vi "exercice5.vi"() -> ()   [LabVIEW 2020]
uses:
  <vilib>/express/express analysis/Spectral/Block/exnSpectralBlock spectral measurements RMS poly.vi
  <vilib>/express/express analysis/Spectral/Block/exnSpectralBlock spectral measurements RMS WFM.vi
  <vilib>/express/express analysis/Spectral/XNode/ExpressSpectralMeasurementsBlockNode.xnode
  <vilib>/measure/NI_MABase.lvlib
panel:
  out "dsa 1st rectangular":cluster{"f0":dbl, "df":dbl, "magnitude":dbl[]}(graph)
  out "dsa 1st hunning":cluster{"f0":dbl, "df":dbl, "magnitude":dbl[]}(graph)
  out "time domain 1st":waveform(dbl)(graph)
  out "k2":dbl
  out "k1":dbl
  out "tw":dbl
  out "freauency resolution":dbl
  in  "N":dbl
  in  "fs":dbl
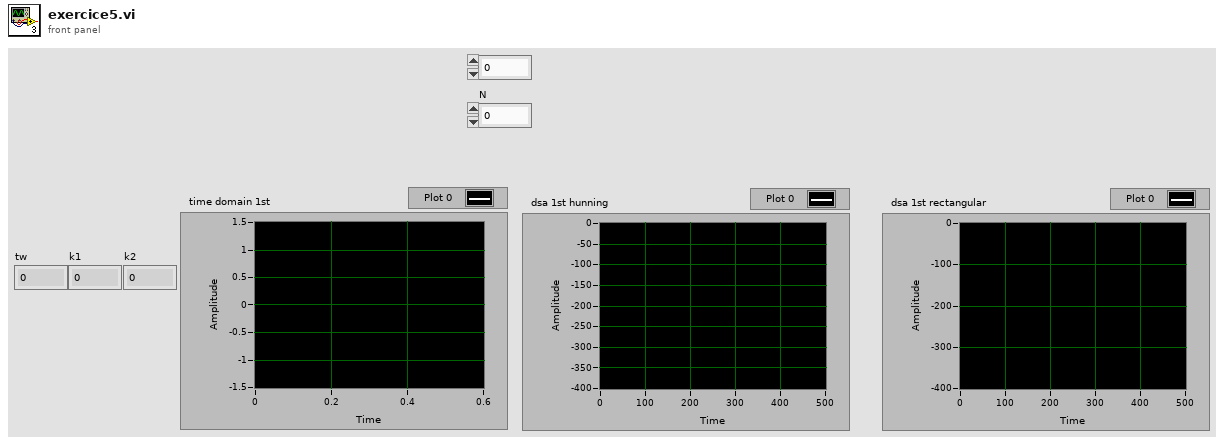
[diagram p1: front panel]
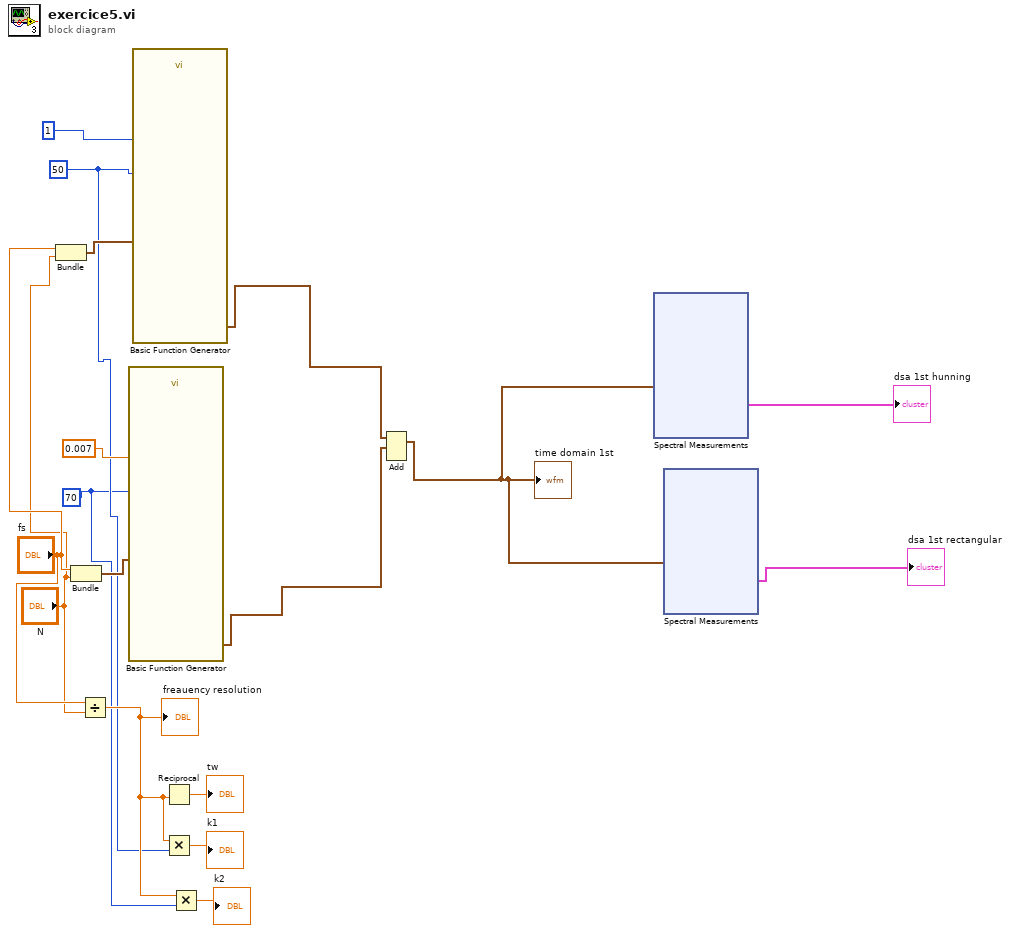
[diagram p0: block diagram]
diagram:
  w7 = 70
  w9 = 50
  n1 = Bundle("fs"="fs", "N"="N") -> (w14:cluster{"fs":dbl, "N":dbl})  [unwired: 1 in]
  n2 = Bundle("fs"="fs", "N"="N") -> (w15:cluster{"fs":dbl, "N":dbl})  [unwired: 1 in]
  n3 = Divide(x="fs", y="N") -> (x/y=w10:dbl)
  "freauency resolution" <- w10
  n4 = call <vilib>:"Basic Function Generator.vi"("sampling info"=w15, "amplitude"=0.007, "frequency"=w7) -> ("signal out"=w2:waveform(dbl))  [unwired: 6 in, 2 out]
  n5 = call <vilib>:"Basic Function Generator.vi"("sampling info"=w14, "amplitude"=1, "frequency"=w9) -> ("signal out"=w3:waveform(dbl))  [unwired: 6 in, 2 out]
  n6 = Reciprocal(x=w10) -> (1/x=→"tw":dbl)
  n7 = Multiply(x=w10, y=w9) -> (x*y=→"k1":dbl)
  n8 = Multiply(x=w10, y=w7) -> (x*y=→"k2":dbl)
  n9 = Add(1:w2, 2:w3) -> (0:w1:waveform(dbl))  [unwired: 1 in, 1 out]
  "time domain 1st" <- w1
  n10 = xnode "Spectral Measurements"("Signals"=w1) -> ("FFT - (RMS)"=→"dsa 1st hunning":cluster{"f0":dbl, "df":dbl, "magnitude":dbl[]})  [unwired: 1 in, 2 out]
  n11 = xnode "Spectral Measurements"("Signals"=w1) -> ("FFT - (RMS)"=→"dsa 1st rectangular":cluster{"f0":dbl, "df":dbl, "magnitude":dbl[]})  [unwired: 1 in, 2 out]
